vi "Statistical Analysis.vi"(8 "error in (no error)":errorcluster, 11 "Graph Data In":T1) -> (0 "error out":errorcluster, 3 "Graph Data Out":T1)   [LabVIEW 2019]
doc: "Computes basic statistics (mean, RMS, min, max, peak to peak and frequency) for each waveform in the input data and outputs annotations."
uses:
  controls/Graph Data.ctl
  <vilib>/Utility/miscctls.llb/LVAnnotationListTypeDef.ctl
  <vilib>/Utility/miscctls.llb/LVCursorListTypeDef.ctl
panel:
  # "(Scroll up to see large data in/out clusters)"
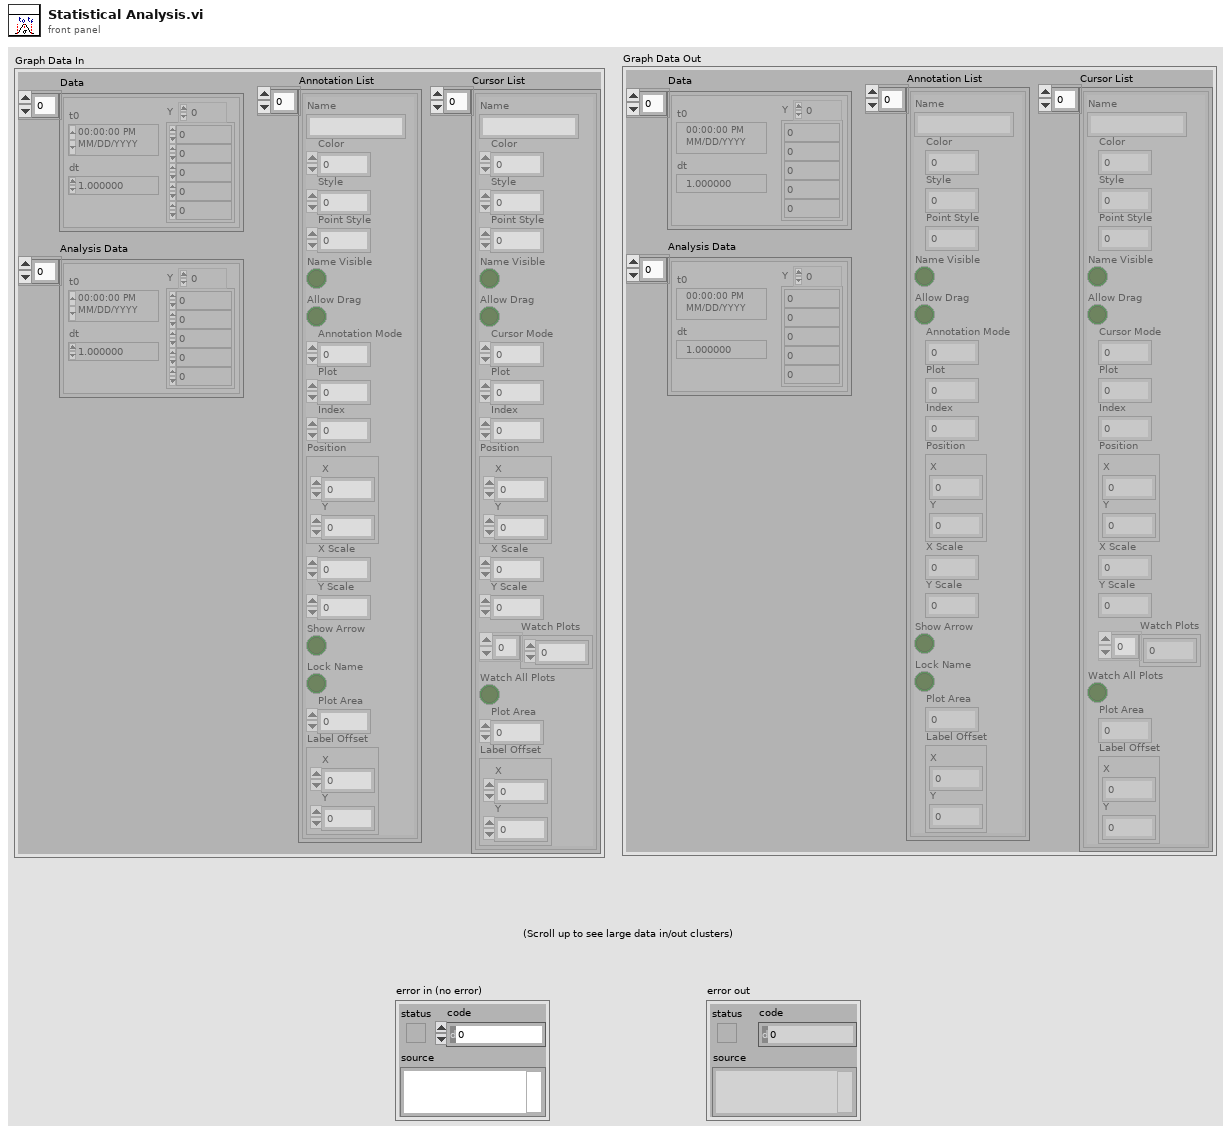
[diagram p1: front panel]
types:
  T1 = typedef "Graph Data.ctl" = cluster{"Data":waveform(dbl)[], "Annotation List":T2, "Cursor List":T3, "Analysis Data":waveform(dbl)[]}
  T2 = typedef "LVAnnotationListTypeDef.ctl" = cluster{"Name":string, "Color":u32, "Style":u8, "Point Style":u8, "Name Visible":bool, "Allow Drag":bool, "Annotation Mode":u32, "Plot":i32, "Index":i32, "Position":cluster{"X":dbl, "Y":dbl}, "X Scale":u32, "Y Scale":u32, "Show Arrow":bool, "Lock Name":bool, "Plot Area":i32, "Label Offset":cluster{"X":dbl, "Y":dbl}}[]
  T3 = typedef "LVCursorListTypeDef.ctl" = cluster{"Name":string, "Color":u32, "Style":u8, "Point Style":u8, "Name Visible":bool, "Allow Drag":bool, "Cursor Mode":u32, "Plot":i32, "Index":i32, "Position":cluster{"X":dbl, "Y":dbl}, "X Scale":u32, "Y Scale":u32, "Watch Plots":i32[], "Watch All Plots":bool, "Plot Area":i32, "Label Offset":cluster{"X":dbl, "Y":dbl}}[]
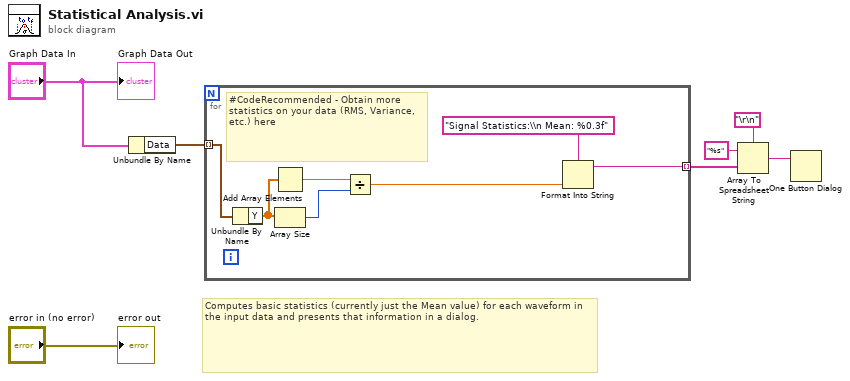
[diagram p0: block diagram]
diagram:
  # "Computes basic statistics (currently just the Mean value) for each waveform in the input data and presents that information in a dialog."
  n1 = Unbundle By Name("Graph Data In") -> ("Data"=w7:waveform(dbl)[])
  n2 = for {
    tunnel: w7 -> [w14] mode=indexing
    tunnel: [w9] -> w4 mode=indexing
    # "#CodeRecommended - Obtain more statistics on your data (RMS, Variance, etc.) here"
    n3 = Unbundle By Name(w14) -> ("Y"=w10:dbl[])
    n4 = Add Array Elements(numeric array=w10) -> (sum=w13:dbl)
    n5 = Array Size(array=w10) -> (size(s)=w11:i32)
    n6 = Divide(x=w13, y=w11) -> (x/y=w12:dbl)
    n7 = Format Into String(format string="Signal Statistics:\\n Mean: %0.3f" ("Signal Statistics"), w12) -> (resulting string=w9:string)  [unwired: 2 in, 1 out]
  }
  n8 = Array To Spreadsheet String(delimiter (Tab)="\r\n", array=w4, 3:"%s" ("format string")) -> (spreadsheet string=w1:string)
  n9 = One Button Dialog(message=w1) -> ()  [unwired: 1 in, 1 out]
  "error out" <- "error in (no error)"
  "Graph Data Out" <- "Graph Data In"
